vi "Calculate Charging Efficiency.vi"(8 "error in (no error)":errorcluster, 9 "T (K)":dbl, 10 "# of charges":i32, 11 "D (m)":dbl) -> (0 "error out":errorcluster, 3 "f":dbl)   [LabVIEW 2015]
doc: "This VI calculates the charging efficiency of a particle as a function of the ambient conditions and the particle size. This VI uses the equation derived by Gunn [1956] for charges greater than two and the approximation developed by Wiedensohler [1988] for charges less than 3. According to Weidensohler [1988], particles smaller than 20 nm can carry at most 1 elementary charge and particles greater than 20 nm and smaller than 70 nm can carry at most 2 elementary charges."
uses:
  Atmospheric/Atmospheric Constants.vi
  Atmospheric/Atmospheric Library.lvlib
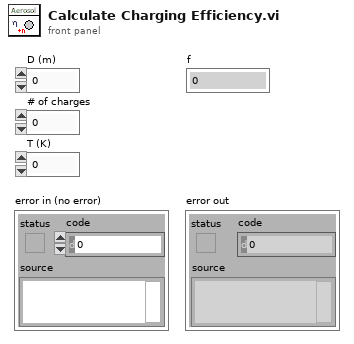
[diagram p1: front panel]
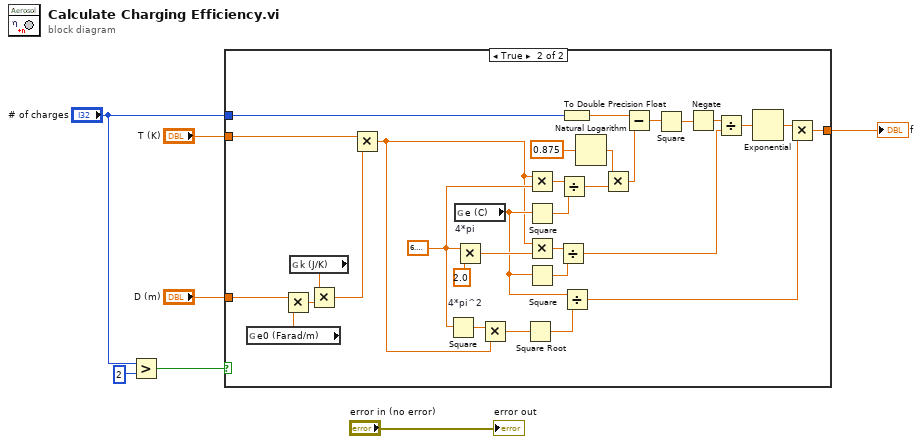
[diagram p0: block diagram]
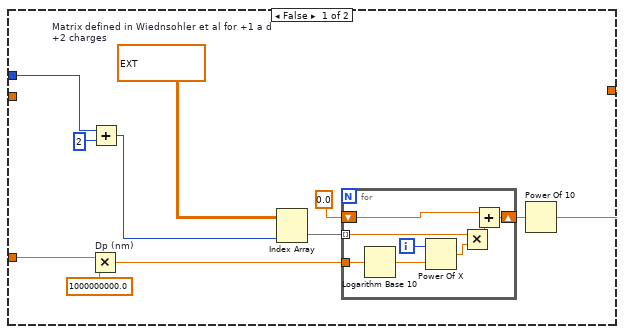
[diagram p2: hidden frame]
diagram:
  n1 = Greater?(x="# of charges", y=2) -> (0:w3:bool)
  n2 = case shown="True" w3 {
    tunnel: "D (m)" -> [w8 w56]
    tunnel: "# of charges" -> [w18 w31]
    tunnel: [w11 w36] -> w4
    tunnel: "T (K)" -> [_ w27]
    frame False {
      w10 = ext[][] [[-26.3328, -2.3197, -0.0003, -2.3484, -44.475599999999999998], [35.9044, 0.6175, -0.1014, 0.6044, 79.3772], [-21.4608, 0.6201, 0.3073, 0.48, -62.89], [7.0867, -0.110500000000000000003, -0.3372, 0.00130000000000000000004, 26.4492], [-1.30880000000000000005, -0.125999999999999999994, 0.102300000000000000003, -0.1553, -5.748], [0.1051, 0.0297, -0.0105, 0.031999999999999999999, 0.5049]]  # Matrix defined in Wiednsohler et al for +1 a d +2 charges
      n3 = Multiply "Dp (nm)"(x=w8, y=1000000000.0) -> (x*y=w16:dbl)
      n4 = Add(x=w18, y=2) -> (x+y=w15:i32)
      n5 = Index Array(array=w10, index (col)=w15) -> (element=w14:ext[])  [unwired: 1 in]
      n6 = for {
        tunnel: w16 -> [w26]
        tunnel: w14 -> [w22] mode=indexing
        shift-right: [w21] -> w12
        shift-left: 0.0 -> [w19]
        i -> [w24]
        n7 = Logarithm Base 10(1:w26) -> (0:w25:dbl)
        n8 = Power Of X(1:w25, 2:w24) -> (0:w23:dbl)
        n9 = Multiply(x=w22, y=w23) -> (x*y=w20:ext)
        n10 = Add(x=w19, y=w20) -> (x+y=w21:ext)
      }
      n11 = Power Of 10(x=w12) -> (10^x=w11:ext)
    }
    frame True {
      w34 = 6.283185307179586
      n12 = global read "Atmospheric Constants.vi" "e0 (Farad/m)"() -> (w54:dbl)
      n13 = Multiply(x=w56, y=w54) -> (x*y=w58:dbl)
      n14 = global read "Atmospheric Constants.vi" "k (J/K)"() -> (w55:dbl)
      n15 = Multiply(x=w55, y=w58) -> (x*y=w57:dbl)
      n16 = Multiply ("Dp*T*k*e0")(x=w27, y=w57) -> (x*y=w32:dbl)
      n17 = Square "4*pi^2"(x=w34) -> (x^2=w33:dbl)
      n18 = global read "Atmospheric Constants.vi" "e (C)"() -> (w35:dbl)
      n19 = Multiply "4*pi"(x=w34, y=2.0) -> (x*y=w43:dbl)
      n20 = Multiply(x=w33, y=w32) -> (x*y=w53:dbl)
      n21 = Square Root(x=w53) -> (sqrt(x)=w37:dbl)
      n22 = Multiply(x=w32, y=w34) -> (x*y=w52:dbl)
      n23 = Square(x=w35) -> (x^2=w51:dbl)
      n24 = Multiply(x=w32, y=w43) -> (x*y=w42:dbl)
      n25 = Square(x=w35) -> (x^2=w41:dbl)
      n26 = Divide(x=w42, y=w41) -> (x/y=w38:dbl)
      n27 = Divide(x=w52, y=w51) -> (x/y=w50:dbl)
      n28 = To Double Precision Float(number=w31) -> (double precision float=w30:dbl)
      n29 = Divide(x=w35, y=w37) -> (x/y=w28:dbl)
      n30 = Natural Logarithm(1:0.875 ("x")) -> (0:w48:dbl)
      n31 = Multiply(x=w48, y=w50) -> (x*y=w47:dbl)
      n32 = Subtract(x=w30, y=w47) -> (x-y=w46:dbl)
      n33 = Square(x=w46) -> (x^2=w45:dbl)
      n34 = Negate(x=w45) -> (-x=w39:dbl)
      n35 = Divide(x=w39, y=w38) -> (x/y=w40:dbl)
      n36 = Exponential(1:w40) -> (0:w29:dbl)
      n37 = Multiply(x=w29, y=w28) -> (x*y=w36:dbl)
    }
  }
  "f" <- w4
  "error out" <- "error in (no error)"
